vi "Write Data.vi"(0 "TCP Socket in":refnum<class "Socket Communication.lvclass">, 1 "data":string, 5 "error in (no error)":errorcluster) -> (14 "TCP Socket out":refnum<class "Socket Communication.lvclass">, 19 "error out":errorcluster)   [LabVIEW 2019, in "Socket Communication.lvclass"]
uses:
  Socket Communication.lvclass
  Socket Communication.lvclass/Socket Communication.ctl
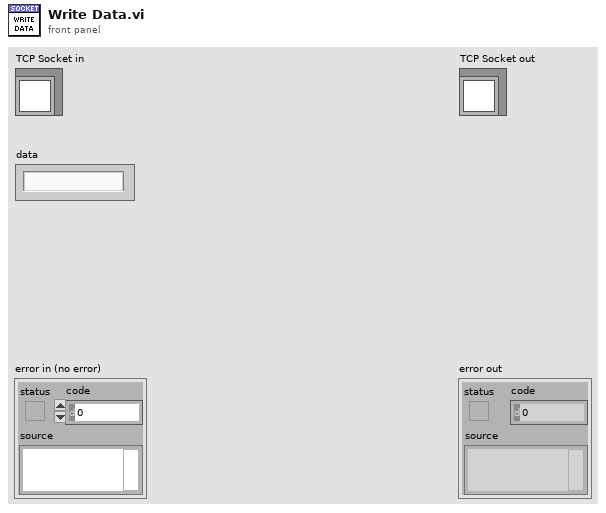
[diagram p1: front panel]
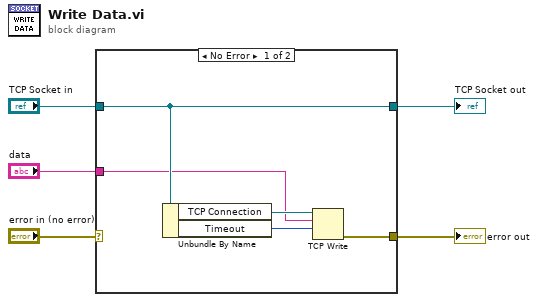
[diagram p0: block diagram]
diagram:
  n1 = case shown="No Error" "error in (no error)" {
    selector: "error in (no error)" -> [_ w12]
    tunnel: [w9 w12] -> w4
    tunnel: [w8 w11] -> w2
    tunnel: "TCP Socket in" -> [w8 w11]
    tunnel: "data" -> [w6 _]
    frame No Error {
      n2 = Unbundle By Name(w8) -> ("TCP Connection"=w10:refnum<k5>, "Timeout"=w7:i32)
      n3 = TCP Write(connection ID=w10, data in=w6, 9:w7) -> (error out=w9:errorcluster)  [unwired: 1 in, 2 out]
    }
    frame Error {
    }
  }
  "error out" <- w4
  "TCP Socket out" <- w2
